vi "Check Is Helper Already Running (Get Queue).vi"(7 "Create? (F: Check)":bool, 11 "GObject in":refnum<vi>) -> (2 "is Running?":bool)   [LabVIEW 2020]
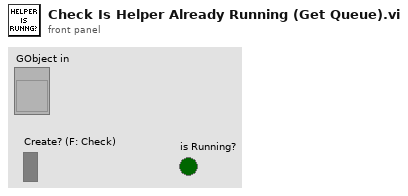
[diagram p1: front panel]
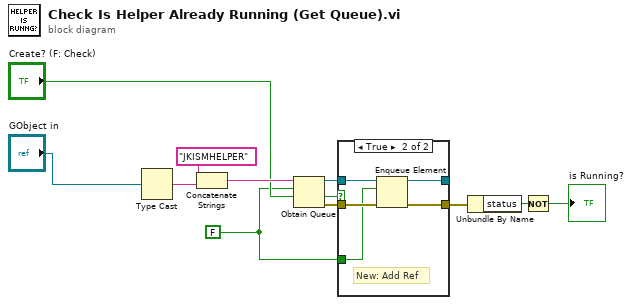
[diagram p0: block diagram]
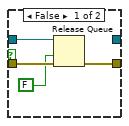
[diagram p2: hidden frame]
diagram:
  w2 = FALSE
  n1 = Type Cast(x="GObject in") -> (*(type *) &x=w10:string)  [unwired: 1 in]
  n2 = Concatenate Strings("JKISMHELPER" ("string"), w10) -> (w12:string)
  n3 = Obtain Queue(name (unnamed)=w12, element data type=w2, create if not found? (T)="Create? (F: Check)") -> (queue out=w5:refnum<queue>, created new?=w6:bool, error out=w3:errorcluster)  [unwired: 2 in]
  n4 = case shown="True" w6 {
    tunnel: w5 -> [w16 w21]
    tunnel: w2 -> [_ w17]
    tunnel: [_ w20] -> _
    tunnel: [w14 w19] -> w4
    tunnel: w3 -> [w15 w18]
    frame False {
      n5 = Release Queue(queue=w16, force destroy? (F)=FALSE, error in (no error)=w15) -> (error out=w14:errorcluster)  [unwired: 2 out]
    }
    frame True {
      # "New: Add Ref"
      n6 = Enqueue Element(queue=w21, element=w17, error in (no error)=w18) -> (queue out=w20:refnum<queue>, error out=w19:errorcluster)  [unwired: 1 in, 1 out]
    }
  }
  n7 = Unbundle By Name(w4) -> ("status"=w8:bool)
  n8 = Not(x=w8) -> (.not. x?=→"is Running?":bool)
